vi "MDAQ_Parse.vi"(8 "error in":errorcluster, 9 "?":T1 {"GATESTOP" format="%04x"; "GATESTRT" format="%04x"; "AMPLITUDE" format="%04x"; "M_CYCLES" format="%04x"; "N_CYCLES" format="%04x"; "STEP" format="%04x"; "BASE" format="%04x"; "CHAN" format="%04x"}, 10 "input buffer":string) -> (0 "error out":errorcluster, 1 "output cluster":T1 {"GATESTOP" format="%04x"; "GATESTRT" format="%04x"; "AMPLITUDE" format="%04x"; "M_CYCLES" format="%04x"; "N_CYCLES" format="%04x"; "STEP" format="%04x"; "BASE" format="%04x"; "CHAN" format="%04x"})   [LabVIEW 2021]
uses:
  Status_Cluster.ctl
  <vilib>/regexp/Match Regular Expression.xnode
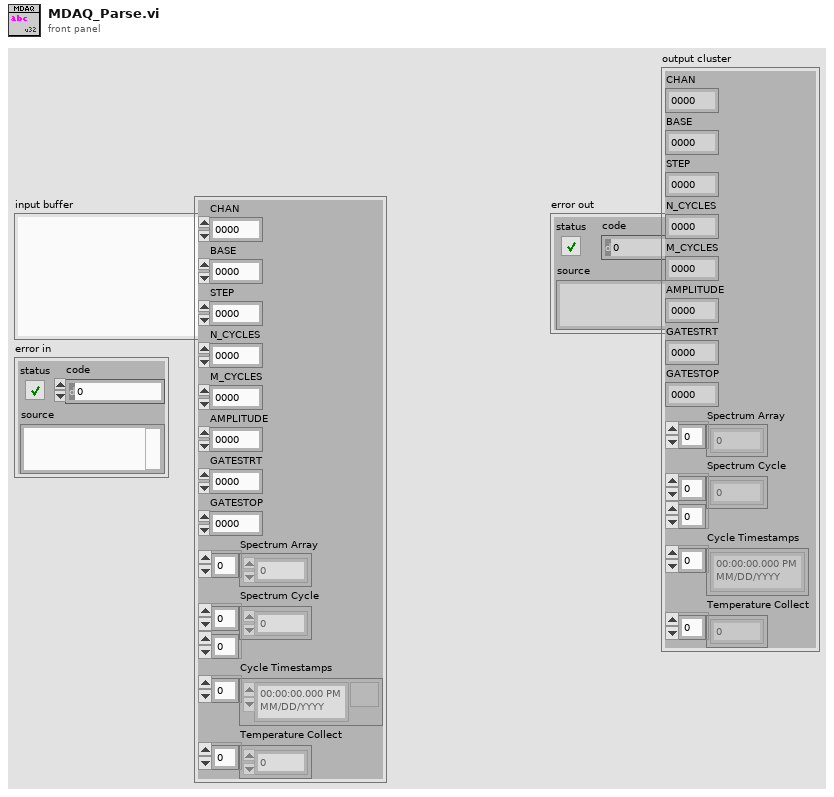
[diagram p1: front panel]
types:
  T1 = typedef "Status_Cluster.ctl" = cluster{"CHAN":u32, "BASE":u32, "STEP":u32, "N_CYCLES":u32, "M_CYCLES":u32, "AMPLITUDE":u32, "GATESTRT":u32, "GATESTOP":u32, "Spectrum Array":u32[], "Spectrum Cycle":u32[][], "Cycle Timestamps":timestamp[], "Temperature Collect":dbl[]}
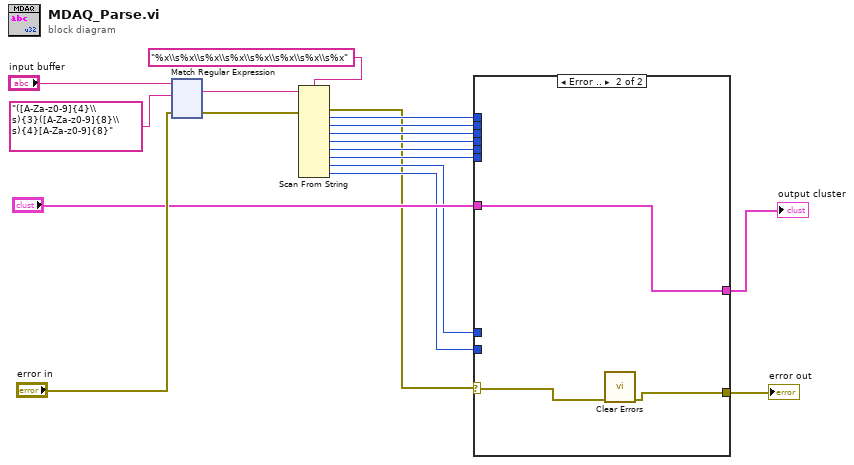
[diagram p0: block diagram]
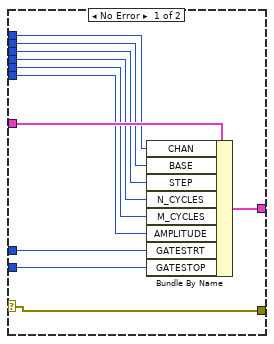
[diagram p2: hidden frame]
diagram:
  n1 = xnode "Match Regular Expression"("input string"="input buffer", "regular expression"="([A-Za-z0-9]{4}\\s){3}([A-Za-z0-9]{8}\\s){4}[A-Za-z0-9]{8}", "error in"="error in") -> ("whole match"=w15:string, "error out"=w14:errorcluster)  [unwired: 3 in, 3 out]
  n2 = Scan From String(format string="%x\\s%x\\s%x\\s%x\\s%x\\s%x\\s%x\\s%x", input string=w15, error in=w14) -> (error out=w2:errorcluster, output 1=w11:u32, output 2=w10:u32, output 3=w9:u32, output 4=w8:u32, output 5=w7:u32, output 6=w6:u32, output 7=w5:u32, output 8=w4:u32)  [unwired: 9 in, 2 out]
  n3 = case shown="Error .." w2 {
    selector: w2 -> [w19 w31]
    tunnel: "?" -> [w29 w32]
    tunnel: w11 -> [w28 _]
    tunnel: w10 -> [w27 _]
    tunnel: w9 -> [w26 _]
    tunnel: w8 -> [w25 _]
    tunnel: w7 -> [w24 _]
    tunnel: w6 -> [w23 _]
    tunnel: w5 -> [w22 _]
    tunnel: w4 -> [w21 _]
    tunnel: [w20 w32] -> w3
    tunnel: [w19 w30] -> w1
    frame No Error {
      n4 = Bundle By Name(cluster=w29, "CHAN"=w28, "BASE"=w27, "STEP"=w26, "N_CYCLES"=w25, "M_CYCLES"=w24, "AMPLITUDE"=w23, "GATESTRT"=w22, "GATESTOP"=w21) -> (w20:T1)
    }
    frame Error {
      n5 = call <vilib>:"Clear Errors.vi"("error in (no error)"=w31) -> ("error out"=w30:errorcluster)  [unwired: 5 in, 1 out]
    }
  }
  "error out" <- w1
  "output cluster" <- w3
